vi "Sound__Acquire_Data_and_Write_to_File.vi"() -> ()   [LabVIEW 2020]
uses:
  <vilib>/sound2/lvsound2.llb/Sampling Mode.ctl
  <vilib>/sound2/lvsound2.llb/Sound Data Format.ctl
  <vilib>/sound2/lvsound2.llb/Sound File Write Open.vi
  <vilib>/sound2/lvsound2.llb/Sound Input Read (DBL).vi
  <vilib>/sound2/lvsound2.llb/Sound File Write (DBL).vi
panel:
  out "Sound Waveform - Channel 2":waveform(dbl)(graph)
  in  "Stop":bool
  out "Sound Waveform - Channel 1":waveform(dbl)(graph)
  out "WAV File Path":path
  in  "Device ID":u32
  # "Acquire Sound Data and Write to File"
  # "Auther: Suparat Yeamkuan\nOverview: Acquire sound from computer microphone and write to WAV file.\nRequirements: Microphone"
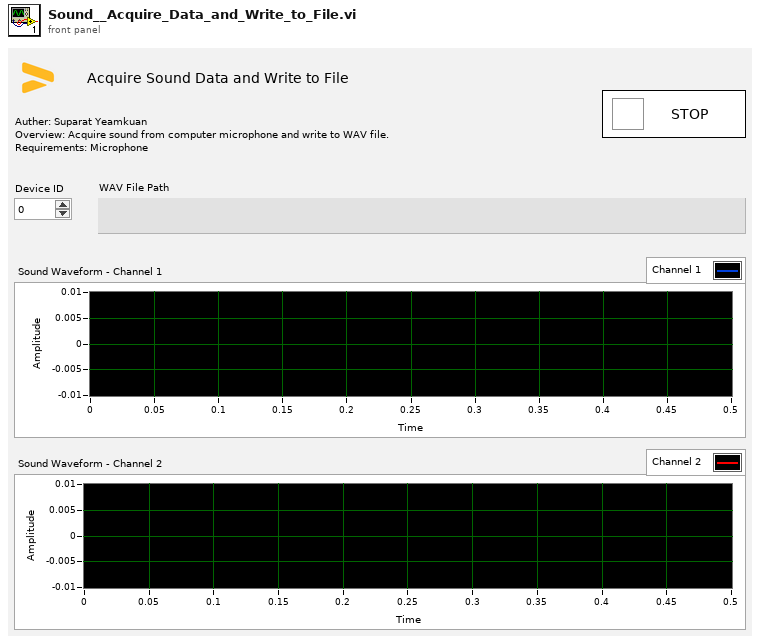
[diagram p1: front panel]
types:
  T1 = typedef "Sound Data Format.ctl" = cluster{"sample rate (S/s)":dbl, "number of channels":i32, "bits per sample":i32}
  T2 = typedef "Sampling Mode.ctl" = i32
  T3 = typedef "Sound File Refnum.ctl" = refnum<file>
  T4 = typedef "Sound Input Task ID.ctl" = u32
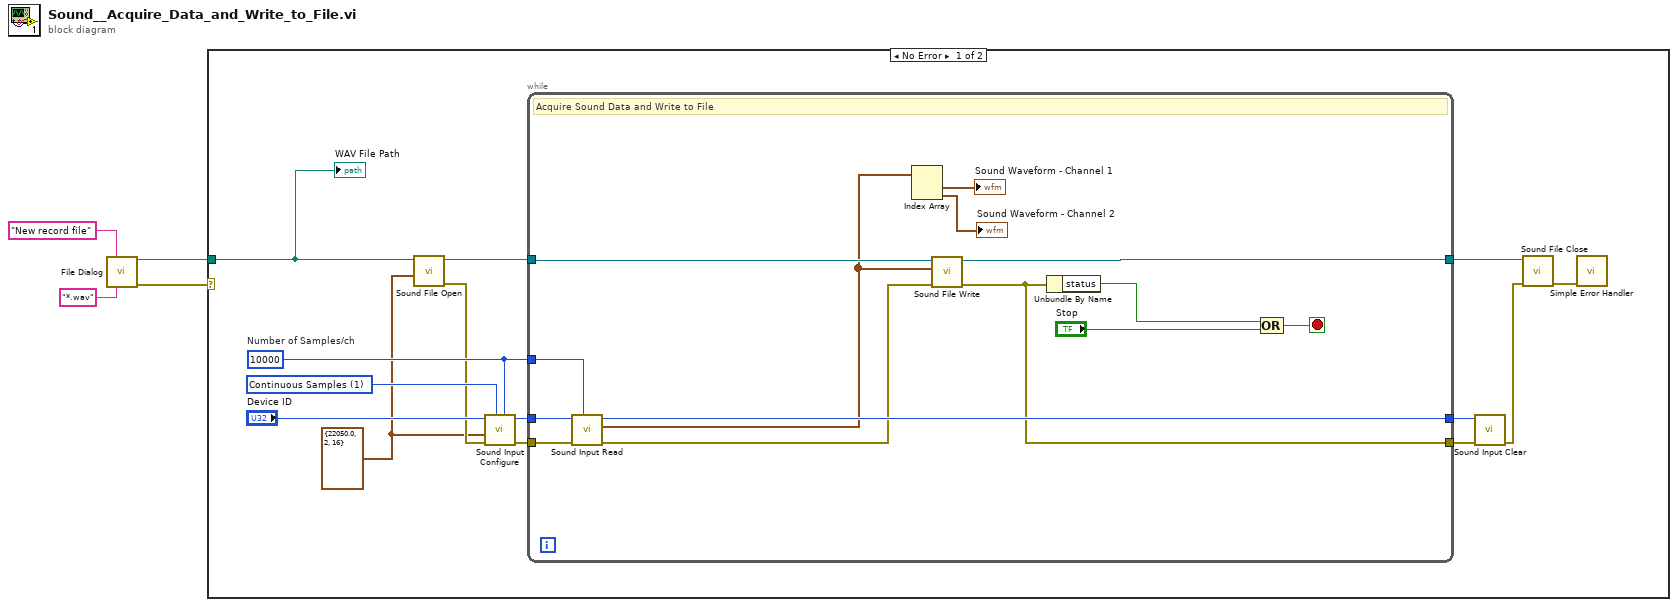
[diagram p0: block diagram]
diagram:
  n1 = call "File Dialog"("prompt"="New record file", "pattern (all files)"="*.wav") -> ("selected path"=w4:path, "error out"=w1:errorcluster)  [unwired: 10 in, 2 out]
  n2 = case shown="No Error" w1 {
    tunnel: w4 -> [w5 _]
    frame No Error {
      w6 = T1 {"sample rate (S/s)"=22050.0, "number of channels"=2, "bits per sample"=16} ("Sound Format")
      w13 = 10000  # Number of Samples/ch
      w12 = T2 1 items=["Finite Samples", "Continuous Samples"] ("sample mode")
      n3 = call-poly <vilib>:"Sound File Open.vi"("sound format"=w6, "path"=w5) -> ("error out"=w8:errorcluster, "sound file refnum"=w11:T3)  [unwired: 8 in]
      n4 = call <vilib>:"Sound Input Configure.vi"("number of samples/ch"=w13, "sample mode"=w12, "error in (no error)"=w8, "sound format"=w6, "device ID"="Device ID") -> ("error out"=w18:errorcluster, "task ID"=w16:T4)  [unwired: 5 in]
      n5 = while {
        tunnel: w13 -> [w29]
        tunnel: w11 -> [w27]
        tunnel: [w26] -> w10
        tunnel: w16 -> [w31]
        tunnel: [w30] -> w15
        tunnel: w18 -> [w32]
        tunnel: [w24] -> w14
        stop <- w28 stop-if-true
        # "Acquire Sound Data and Write to File"
        n6 = call-poly <vilib>:"Sound Input Read.vi"("number of samples/ch"=w29, "error in (no error)"=w32, "task ID"=w31) -> ("error out"=w25:errorcluster, "data"=w21:waveform(dbl)[], "task ID out"=w30:T4)  [unwired: 6 in]
        n7 = Index Array(array=w21) -> (element #1=→"Sound Waveform - Channel 1":waveform(dbl), element #2=→"Sound Waveform - Channel 2":waveform(dbl))  [unwired: 2 in]
        n8 = call-poly <vilib>:"Sound File Write.vi"("error in (no error)"=w25, "data"=w21, "sound file refnum"=w27) -> ("error out"=w24:errorcluster, "sound file refnum out"=w26:T3)  [unwired: 7 in]
        n9 = Unbundle By Name(w24) -> ("status"=w23:bool)
        n10 = Compound Arithmetic op=OR(w23, "Stop") -> (w28:bool)
      }
      n11 = call <vilib>:"Sound Input Clear.vi"("error in (no error)"=w14, "task ID"=w15) -> ("error out"=w9:errorcluster)  [unwired: 9 in]
      n12 = call <vilib>:"Sound File Close.vi"("error in (no error)"=w9, "sound file refnum"=w10) -> ("error out"=w7:errorcluster)  [unwired: 9 in]
      n13 = call <vilib>:"Simple Error Handler.vi"("error in (no error)"=w7) -> ()  [unwired: 4 in, 5 out]
      "WAV File Path" <- w5
    }
    frame Error {
    }
  }
